vi "CallByRefParallel Is running.vi"(8 "error in (no error)":errorcluster, 11 "VI Refnum":refnum<vi>) -> (0 "error out":errorcluster, 2 "Is running?":bool, 3 "VI Refnum dup":refnum<vi>)   [LabVIEW 2014, in "COSYLib.lvlib"]
doc: "Utility VI to check if a dynamically called VI (using \"CallByRefParallel\") is (still) running."
uses:
  COSYLib.lvlib
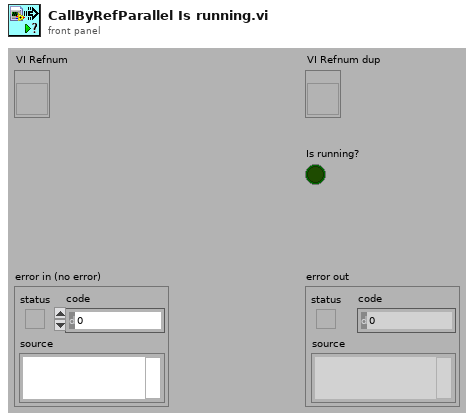
[diagram p1: front panel]
types:
  T1 = enum32{"Bad", "Idle", "Run top level", "Running"}
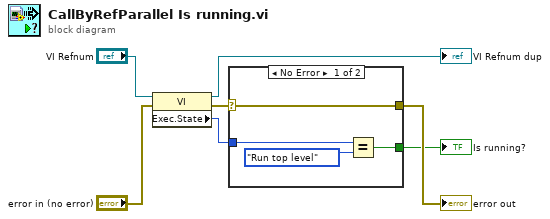
[diagram p0: block diagram]
diagram:
  n1 = property class="VI"(reference="VI Refnum", error in="error in (no error)") -> (reference out=→"VI Refnum dup":refnum<vi>, error out=w5:errorcluster, "Exec.State"=w4:T1)
  n2 = case shown="No Error" w5 {
    selector: w5 -> [w11 w12]
    tunnel: w4 -> [w10 _]
    tunnel: [w11 w12] -> w2
    tunnel: [w8 _] -> w1
    frame No Error {
      n3 = Equal?(x=w10, y=T1."Run top level") -> (x = y?=w8:bool)
    }
    frame Error {
    }
  }
  "error out" <- w2
  "Is running?" <- w1
